vi "Write TDMS.vi"(8 "error in (no error)":errorcluster, 10 "TDMS":refnum<k34>, 11 "PluginInterface in":refnum<class "PluginInterface.lvclass">) -> (0 "error out":errorcluster, 3 "PluginInterface out":refnum<class "PluginInterface.lvclass">)   [LabVIEW 2013, in "PluginInterface.lvlib" / "PluginInterface.lvclass"]
uses:
  PluginInterface.lvclass
  PluginInterface.lvclass/PluginInterface.ctl
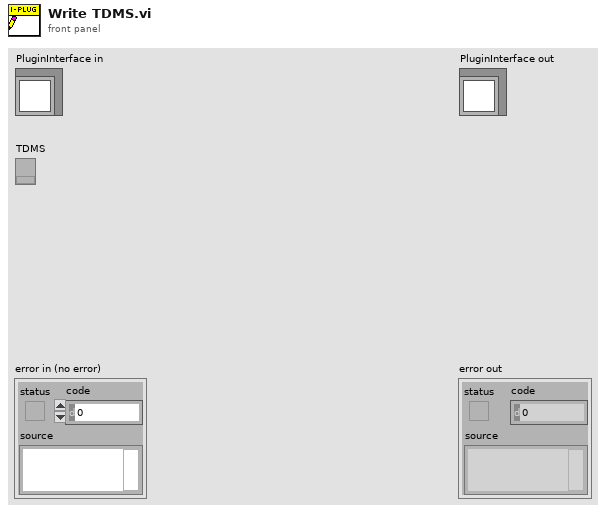
[diagram p1: front panel]
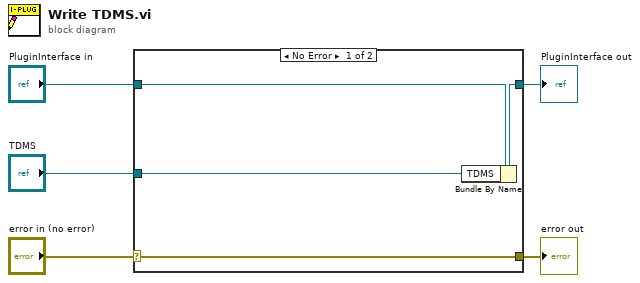
[diagram p0: block diagram]
diagram:
  n1 = case shown="No Error" "error in (no error)" {
    selector: "error in (no error)" -> [w9 w10]
    tunnel: [w9 w10] -> w4
    tunnel: [w7 w11] -> w2
    tunnel: "PluginInterface in" -> [w8 w11]
    tunnel: "TDMS" -> [w6 _]
    frame No Error {
      n2 = Bundle By Name(cluster=w8, "TDMS"=w6) -> (w7:refnum<class "PluginInterface.lvclass">)
    }
    frame Error {
    }
  }
  "error out" <- w4
  "PluginInterface out" <- w2
